vi "5 Balls.vi"() -> ()   [LabVIEW 2020]
uses:
  Controls/Autonomo/Autonomous5BallStates.ctl
  Global Variable/Trajectory Variables.vi
  Global Variable/Actuators_N_Sensors.vi
panel:
  out "AtReference":bool
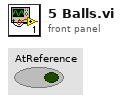
[diagram p1: front panel]
types:
  T1 = typedef "Autonomous5BallStates.ctl" = enum16{"Reset", "Trajectory 1", "Reset Encoder", "Trajectory 2", "Shoot 1", "Reset Encoder 1", "Trajectory 3", "Shoot 2", "Reset Encoder 2", "Trajectory 4", "Reset Encoder 3", "Trajectory 5", "Shoot 3", "Finish"}
  T2 = typedef "Trajectory_Library.lvlib/TRAJ_STATE.ctl" = cluster{"TimeSeconds":dbl, "Velocity":dbl, "Acceleration":dbl, "POSE":T3, "Curvature":dbl}
  T3 = typedef "Trajectory_Library.lvlib/POSE2D.ctl" = cluster{"TRANSLATION":T4, "ROTATION":T5}
  T4 = typedef "Trajectory_Library.lvlib/TRANSLATION2D.ctl" = cluster{"X":dbl, "Y":dbl}
  T5 = typedef "Trajectory_Library.lvlib/ROTATION2D.ctl" = cluster{"VALUE":dbl, "COS":dbl, "SIN":dbl}
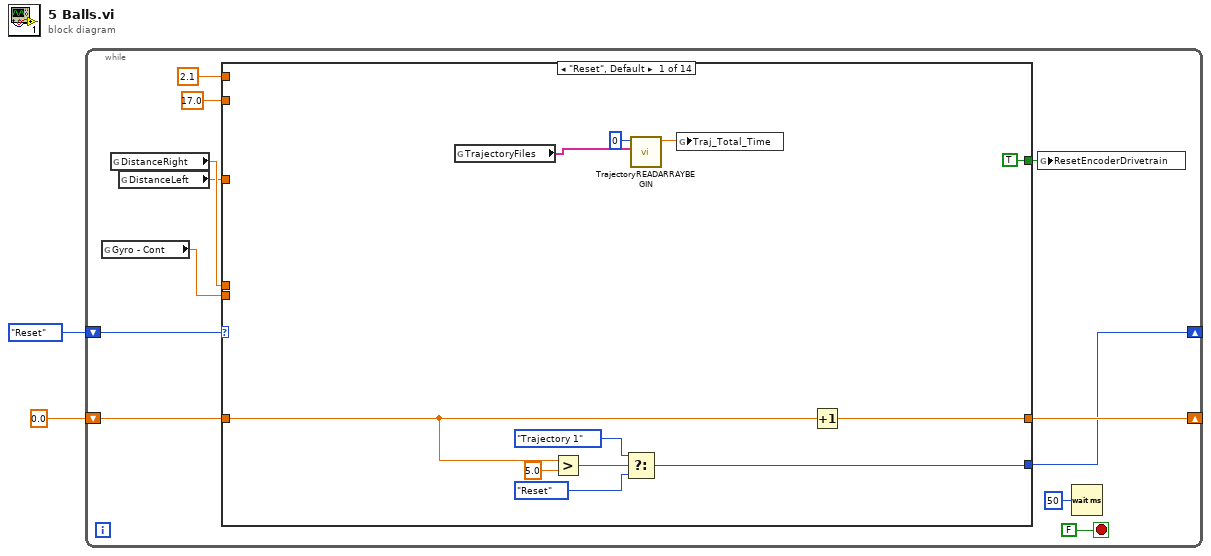
[diagram p0: block diagram]
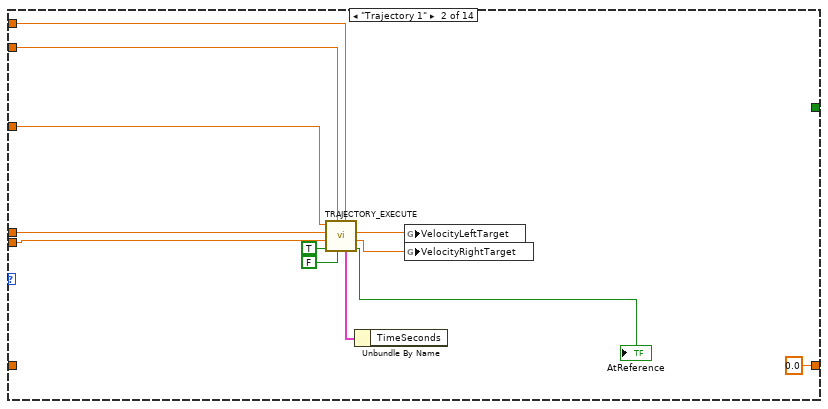
[diagram p2: hidden frame]
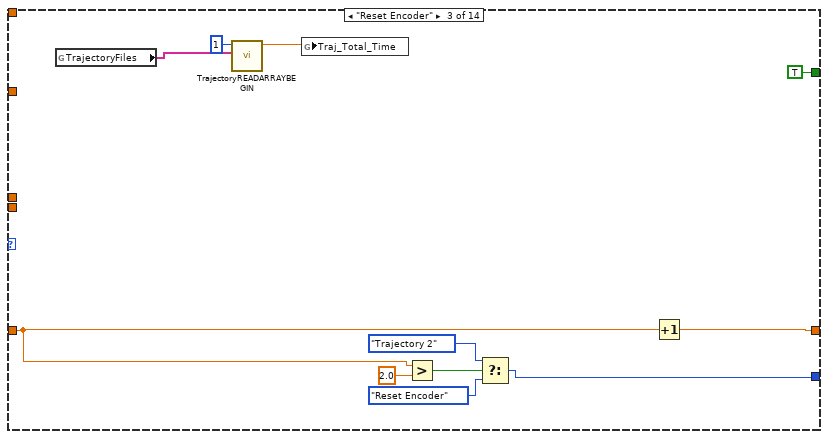
[diagram p3: hidden frame]
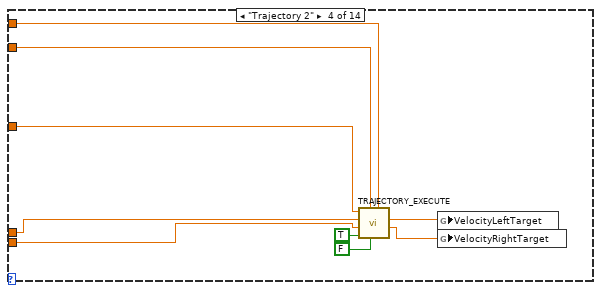
[diagram p4: hidden frame]
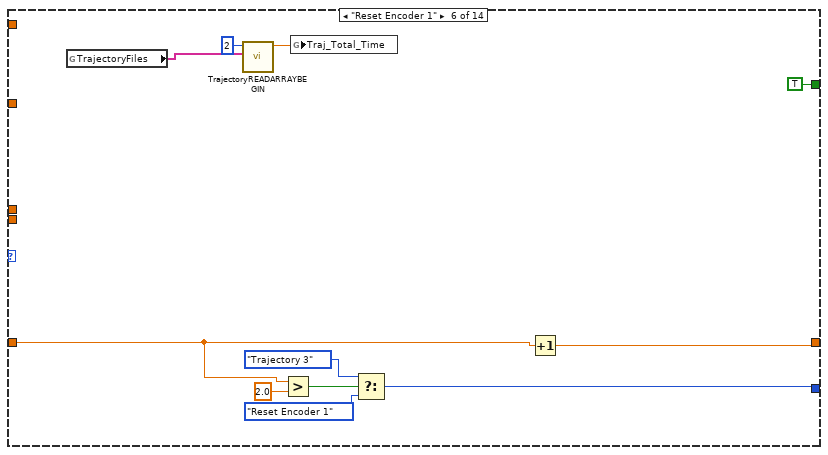
[diagram p6: hidden frame]
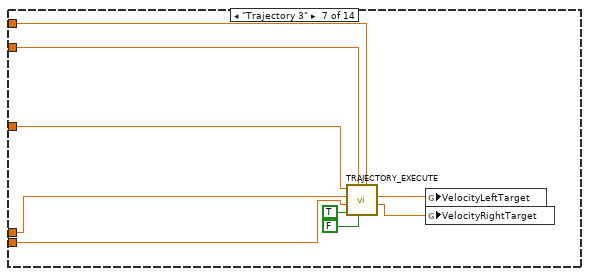
[diagram p7: hidden frame]
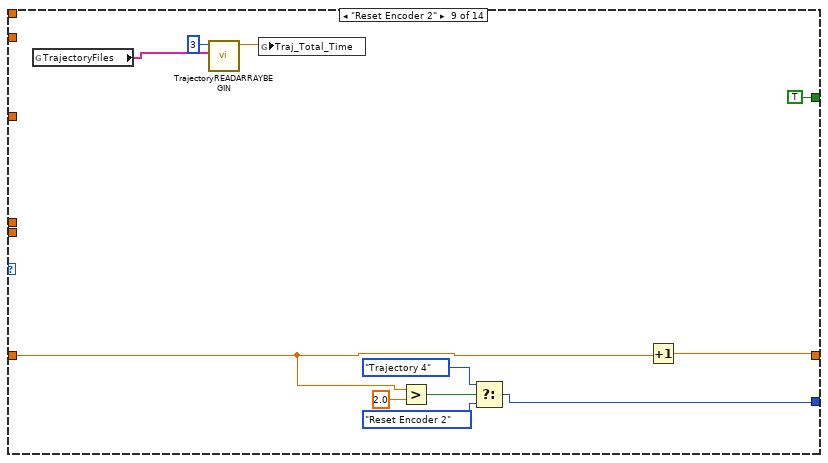
[diagram p9: hidden frame]
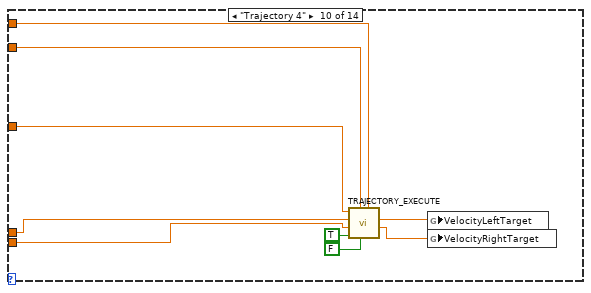
[diagram p10: hidden frame]
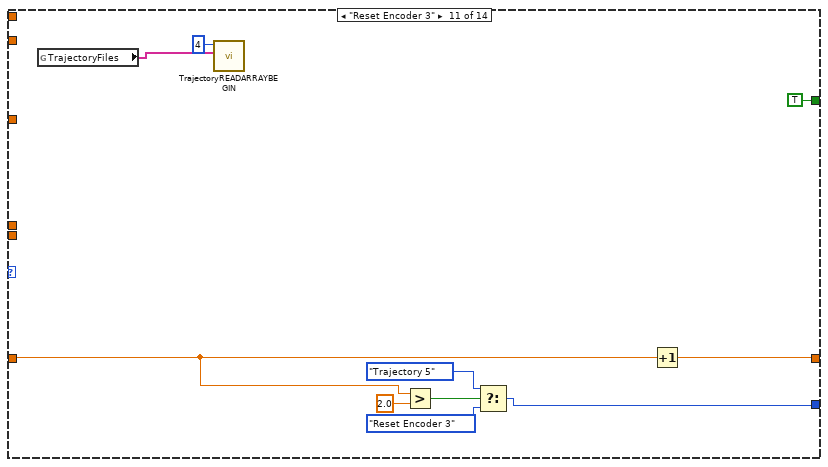
[diagram p11: hidden frame]
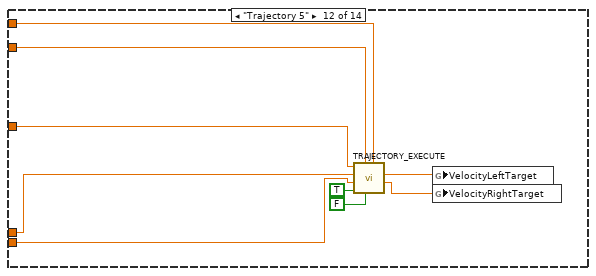
[diagram p12: hidden frame]
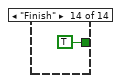
[diagram p14: hidden frame]
diagram:
  n1 = while {
    shift-right: [w9] -> _
    shift-left: Autonomous5BallStates."Reset" ("States 5 Ball") -> [w12]
    shift-right: [w10] -> _
    shift-left: 0.0 ("y") -> [w11]
    stop <- FALSE stop-if-true
    n2 = global read "Actuators_N_Sensors.vi" "Gyro - Cont"() -> (w4:dbl)
    n3 = global read "Trajectory Variables.vi" "DistanceRight"() -> (w8:dbl)
    n4 = global read "Trajectory Variables.vi" "DistanceLeft"() -> (w7:dbl)
    n5 = case shown="\"Reset\", Default" w12 {
      tunnel: w11 -> [w24 _ w42 _ _ w59 _ _ w79 _ w98 _ _ _]
      tunnel: [w16 0.0 ("y") w39 _ _ w60 _ _ w80 _ w99 _ _ _] -> w10
      tunnel: [w20 _ w41 _ _ w61 _ _ w81 _ w100 _ _ _] -> w9
      tunnel: w8 -> [_ w37 _ w50 _ _ w70 _ _ w90 _ w109 _ _]
      tunnel: w7 -> [_ w36 _ w51 _ _ w71 _ _ w91 _ w110 _ _]
      tunnel: 17.0 ("Max Speed\nFT/SEC") -> [_ w35 _ w52 _ _ w73 _ _ w92 _ w111 _ _]
      tunnel: 2.1 ("Track Width FT") -> [_ w34 _ w53 _ _ w72 _ _ w93 _ w112 _ _]
      tunnel: w4 -> [_ w33 _ w49 _ _ w69 _ _ w89 _ w108 _ _]
      tunnel: [TRUE ("ResetEncoderDrivetrain") _ TRUE ("ResetEncoderDrivetrain") _ _ TRUE ("ResetEncoderDrivetrain") _ _ TRUE ("ResetEncoderDrivetrain") _ TRUE ("ResetEncoderDrivetrain") _ _ TRUE ("ResetEncoderDrivetrain")] -> w3
      frame "Reset", Default {
        n6 = global read "Trajectory Variables.vi" "TrajectoryFiles"() -> (w18:string[])
        n7 = Greater?(x=w24, y=5.0) -> (0:w23:bool)
        n8 = Select(t=Autonomous5BallStates."Trajectory 1" ("States 5 Ball"), s=w23, f=Autonomous5BallStates."Reset" ("States 5 Ball")) -> (s? t:f=w20:T1)
        n9 = call "TrajectoryREADARRAYBEGIN.vi"("Trajectories Files"=w18, "Trajectory Number 0-x"=0) -> ("TotalTImeSecs"=w15:dbl)  [unwired: 8 in, 1 out]
        n10 = global write "Trajectory Variables.vi" "Traj_Total_Time"(w15) -> ()
        n11 = Increment(x=w24) -> (x+1=w16:dbl)
      }
      frame "Trajectory 1" {
        n12 = call "TRAJECTORY_EXECUTE.vi"("Track Width FT"=w34, "RamseteEnable"=FALSE, "Max Speed\nFT/SEC"=w35, "Init"=TRUE, "Gyro Continous\n (inc counterclockwise)"=w33, "Right Distance"=w37, "Left Distance"=w36) -> ("AtReference"=→"AtReference":bool, "Right Speed Target"=w30:dbl, "Left Speed Target"=w31:dbl, "OutputTRAJ_STATE (SI)"=w26:T2)  [unwired: 1 out]
        n13 = Unbundle By Name(w26) -> ()  [unwired: 1 out]
        n14 = global write "Trajectory Variables.vi" "VelocityLeftTarget"(w31) -> ()
        n15 = global write "Trajectory Variables.vi" "VelocityRightTarget"(w30) -> ()
      }
      frame "Reset Encoder" {
        n16 = global read "Trajectory Variables.vi" "TrajectoryFiles"() -> (w48:string[])
        n17 = call "TrajectoryREADARRAYBEGIN.vi"("Trajectories Files"=w48, "Trajectory Number 0-x"=1) -> ("TotalTImeSecs"=w38:dbl)  [unwired: 8 in, 1 out]
        n18 = global write "Trajectory Variables.vi" "Traj_Total_Time"(w38) -> ()
        n19 = Greater?(x=w42, y=2.0) -> (0:w45:bool)
        n20 = Select(t=Autonomous5BallStates."Trajectory 2" ("States 5 Ball"), s=w45, f=Autonomous5BallStates."Reset Encoder" ("States 5 Ball")) -> (s? t:f=w41:T1)
        n21 = Increment(x=w42) -> (x+1=w39:dbl)
      }
      frame "Trajectory 2" {
        n22 = call "TRAJECTORY_EXECUTE.vi"("Track Width FT"=w53, "RamseteEnable"=FALSE, "Max Speed\nFT/SEC"=w52, "Init"=TRUE, "Gyro Continous\n (inc counterclockwise)"=w49, "Right Distance"=w50, "Left Distance"=w51) -> ("Right Speed Target"=w57:dbl, "Left Speed Target"=w56:dbl)  [unwired: 3 out]
        n23 = global write "Trajectory Variables.vi" "VelocityLeftTarget"(w56) -> ()
        n24 = global write "Trajectory Variables.vi" "VelocityRightTarget"(w57) -> ()
      }
      frame "Shoot 1" {
      }
      frame "Reset Encoder 1" {
        n25 = global read "Trajectory Variables.vi" "TrajectoryFiles"() -> (w68:string[])
        n26 = call "TrajectoryREADARRAYBEGIN.vi"("Trajectories Files"=w68, "Trajectory Number 0-x"=2) -> ("TotalTImeSecs"=w58:dbl)  [unwired: 8 in, 1 out]
        n27 = Greater?(x=w59, y=2.0) -> (0:w65:bool)
        n28 = global write "Trajectory Variables.vi" "Traj_Total_Time"(w58) -> ()
        n29 = Select(t=Autonomous5BallStates."Trajectory 3" ("States 5 Ball"), s=w65, f=Autonomous5BallStates."Reset Encoder 1" ("States 5 Ball")) -> (s? t:f=w61:T1)
        n30 = Increment(x=w59) -> (x+1=w60:dbl)
      }
      frame "Trajectory 3" {
        n31 = call "TRAJECTORY_EXECUTE.vi"("Track Width FT"=w72, "RamseteEnable"=FALSE, "Max Speed\nFT/SEC"=w73, "Init"=TRUE, "Gyro Continous\n (inc counterclockwise)"=w69, "Right Distance"=w70, "Left Distance"=w71) -> ("Right Speed Target"=w77:dbl, "Left Speed Target"=w76:dbl)  [unwired: 3 out]
        n32 = global write "Trajectory Variables.vi" "VelocityLeftTarget"(w76) -> ()
        n33 = global write "Trajectory Variables.vi" "VelocityRightTarget"(w77) -> ()
      }
      frame "Shoot 2" {
      }
      frame "Reset Encoder 2" {
        n34 = global read "Trajectory Variables.vi" "TrajectoryFiles"() -> (w88:string[])
        n35 = call "TrajectoryREADARRAYBEGIN.vi"("Trajectories Files"=w88, "Trajectory Number 0-x"=3) -> ("TotalTImeSecs"=w78:dbl)  [unwired: 8 in, 1 out]
        n36 = global write "Trajectory Variables.vi" "Traj_Total_Time"(w78) -> ()
        n37 = Greater?(x=w79, y=2.0) -> (0:w84:bool)
        n38 = Select(t=Autonomous5BallStates."Trajectory 4" ("States 5 Ball"), s=w84, f=Autonomous5BallStates."Reset Encoder 2" ("States 5 Ball")) -> (s? t:f=w81:T1)
        n39 = Increment(x=w79) -> (x+1=w80:dbl)
      }
      frame "Trajectory 4" {
        n40 = call "TRAJECTORY_EXECUTE.vi"("Track Width FT"=w93, "RamseteEnable"=FALSE, "Max Speed\nFT/SEC"=w92, "Init"=TRUE, "Gyro Continous\n (inc counterclockwise)"=w89, "Right Distance"=w90, "Left Distance"=w91) -> ("Right Speed Target"=w97:dbl, "Left Speed Target"=w96:dbl)  [unwired: 3 out]
        n41 = global write "Trajectory Variables.vi" "VelocityLeftTarget"(w96) -> ()
        n42 = global write "Trajectory Variables.vi" "VelocityRightTarget"(w97) -> ()
      }
      frame "Reset Encoder 3" {
        n43 = global read "Trajectory Variables.vi" "TrajectoryFiles"() -> (w107:string[])
        n44 = call "TrajectoryREADARRAYBEGIN.vi"("Trajectories Files"=w107, "Trajectory Number 0-x"=4) -> ()  [unwired: 8 in, 2 out]
        n45 = Greater?(x=w98, y=2.0) -> (0:w103:bool)
        n46 = Select(t=Autonomous5BallStates."Trajectory 5" ("States 5 Ball"), s=w103, f=Autonomous5BallStates."Reset Encoder 3" ("States 5 Ball")) -> (s? t:f=w100:T1)
        n47 = Increment(x=w98) -> (x+1=w99:dbl)
      }
      frame "Trajectory 5" {
        n48 = call "TRAJECTORY_EXECUTE.vi"("Track Width FT"=w112, "RamseteEnable"=FALSE, "Max Speed\nFT/SEC"=w111, "Init"=TRUE, "Gyro Continous\n (inc counterclockwise)"=w108, "Right Distance"=w109, "Left Distance"=w110) -> ("Right Speed Target"=w116:dbl, "Left Speed Target"=w115:dbl)  [unwired: 3 out]
        n49 = global write "Trajectory Variables.vi" "VelocityLeftTarget"(w115) -> ()
        n50 = global write "Trajectory Variables.vi" "VelocityRightTarget"(w116) -> ()
      }
      frame "Shoot 3" {
      }
      frame "Finish" {
      }
    }
    n51 = global write "Actuators_N_Sensors.vi" "ResetEncoderDrivetrain"(w3) -> ()
    n52 = Wait (ms)(milliseconds to wait=u32 50) -> ()  [unwired: 1 out]
  }
